vi "Sensirion Flow Meter Read.vi"() -> ()   [LabVIEW 2014]
panel:
  out "MeasureResult Scaled":dbl
  in  "COMPort":u16=20
  out "Waveform Chart":dbl(graph)
  in  "stop":bool
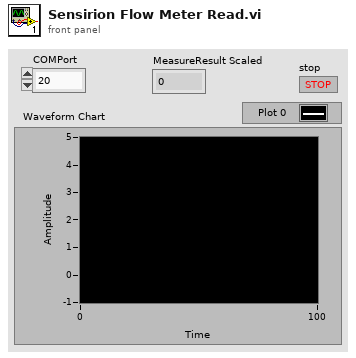
[diagram p1: front panel]
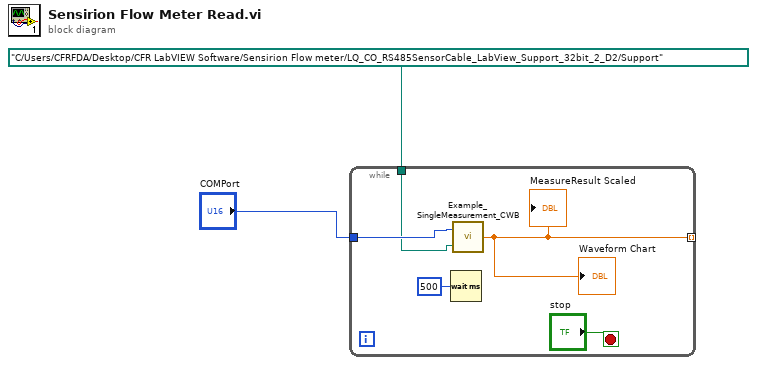
[diagram p0: block diagram]
diagram:
  n1 = while {
    tunnel: [w5] -> _ mode=indexing
    tunnel: "COMPort" -> [w4]
    tunnel: path "C:/Users/CFRFDA/Desktop/CFR LabVIEW Software/Sensirion Flow meter/LQ_CO_RS485SensorCable_LabView_Support_32bit_2_D2/Support" ("base path") -> [w3]
    stop <- "stop" stop-if-true
    n2 = Wait (ms)(milliseconds to wait=u32 500) -> ()  [unwired: 1 out]
    n3 = call "Example_SingleMeasurement_CWB.vi"("base path"=w3, "COMPort"=w4) -> ("MeasureResult Scaled"=w5:dbl)
    "Waveform Chart" <- w5
    "MeasureResult Scaled" <- w5
  }
